vi "Format_append_data.vi"(1 "Numbers to append":dbl[](array[numeric]) format="%#_6f", 2 "Strings without numbers":string[](array[string])) -> (0 "Final Strings":string[](array[string]))   [LabVIEW 2009]
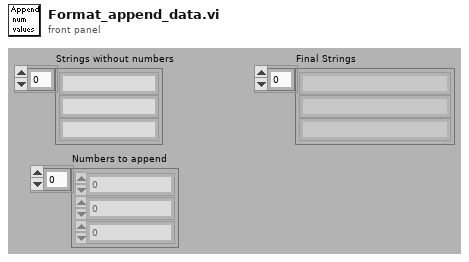
[diagram p1: front panel]
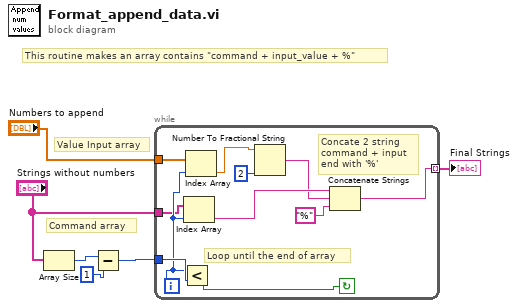
[diagram p0: block diagram]
diagram:
  # "This routine makes an array contains \"command + input_value + %\""
  # "Value Input array"
  # "Command array"
  n1 = Array Size(array="Strings without numbers") -> (size(s)=w6:i32)
  n2 = Subtract(x=w6, y=1) -> (x-y=w2:i32)
  n3 = while {
    tunnel: w2 -> [w16]
    tunnel: "Numbers to append" -> [w15]
    tunnel: "Strings without numbers" -> [w13]
    tunnel: [w8] -> w3 mode=indexing
    i -> [w14]
    stop <- w17 continue-if-true
    # "Loop until the end of array"
    # "Concate 2 string\ncommand + input\nend with '%'"
    n4 = Less?(x=w14, y=w16) -> (x < y?=w17:bool)
    n5 = Index Array(array=w13, index=w14) -> (element=w11:string)
    n6 = Index Array(array=w15, index=w14) -> (element=w12:dbl)
    n7 = Number To Fractional String(number=w12, precision (6)=2) -> (F-format string=w9:string)  [unwired: 2 in]
    n8 = Concatenate Strings(w11, w9, "%" ("Carriage Return Constant")) -> (w8:string)
  }
  "Final Strings" <- w3
